vi "Query Frequency Mode.vi"(8 "error in (no error)":errorcluster, 10 "Channel (0: Channel 1)":T2 items=["Channel 1", "Channel 2"], 11 "VISA resource name":refnum<visa-resource-name>) -> (0 "error out":errorcluster, 1 "Mode (0: CW)":T1, 3 "VISA resource name out":refnum<visa-resource-name>)   [LabVIEW 2015, in "Tektronix AFG 3000 Series.lvlib"]
doc: "Queries the frequency mode (sweep vs. continuous) of a Tektronix AFG 3000 series function generator."
uses:
  Tektronix AFG 3000 Series.lvlib
  controls.llb/Channel.ctl
  controls.llb/Frequency Mode.ctl
  <vilib>/Utility/error.llb/DialogType.ctl
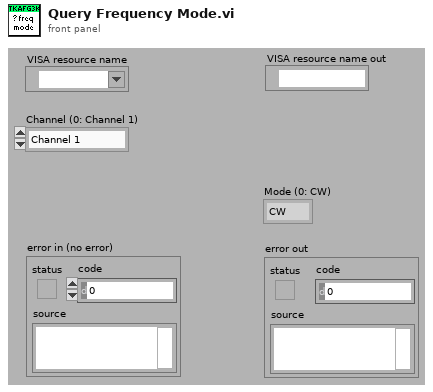
[diagram p1: front panel]
types:
  T1 = typedef "Frequency Mode.ctl" = enum16{"CW", "Sweep"}
  T2 = typedef "Channel.ctl" = u16
  T3 = typedef "DialogType.ctl" = u16
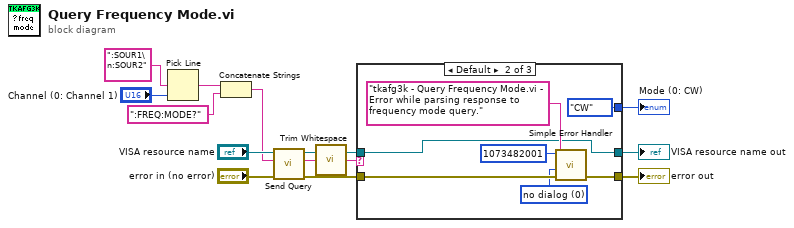
[diagram p0: block diagram]
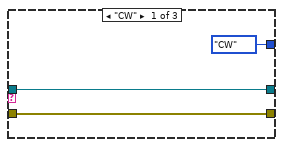
[diagram p2: hidden frame]
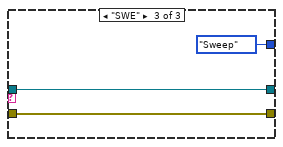
[diagram p3: hidden frame]
diagram:
  n1 = Pick Line(multi-line string=":SOUR1\n:SOUR2", line index="Channel (0: Channel 1)") -> (output string=w11:string)  [unwired: 1 out]
  n2 = Concatenate Strings(w11, ":FREQ:MODE?" ("format string")) -> (w10:string)
  n3 = call "Send Query.vi"("error in (no error)"="error in (no error)", "write buffer"=w10, "VISA resource name"="VISA resource name") -> ("error out"=w6:errorcluster, "read buffer"=w2:string, "VISA resource name out"=w5:refnum<visa-resource-name>)  [unwired: 1 in, 5 out]
  n4 = call <vilib>:"Trim Whitespace.vi"("string"=w2) -> ("trimmed string"=w1:string)  [unwired: 1 in]
  n5 = case shown="Default" w1 {
    tunnel: [Frequency_Mode."CW" ("Mode (0: CW) 2") Frequency_Mode."CW" ("Mode (0: CW) 2") Frequency_Mode."Sweep" ("Mode (0: CW) 2")] -> w7
    tunnel: w6 -> [w15 w23 w25]
    tunnel: w5 -> [w16 w18 w26]
    tunnel: [w16 w18 w26] -> w4
    tunnel: [w15 w22 w25] -> w3
    frame "CW" {
    }
    frame Default {
      w21 = T3 0 items=["no dialog", "OK message", "continue or stop message", "OK message + warnings", "continue/stop + warnings"] ("type of dialog (OK msg:1)")
      n6 = call <vilib>:"Simple Error Handler.vi"("error code (no error:0)"=1073482001, "error source (\" \")"="tkafg3k - Query Frequency Mode.vi - Error while parsing response to frequency mode query." ("error source (\" \")"), "type of dialog (OK msg:1)"=w21, "error in (no error)"=w23) -> ("error out"=w22:errorcluster)  [unwired: 5 out]
    }
    frame "SWE" {
    }
  }
  "error out" <- w3
  "VISA resource name out" <- w4
  "Mode (0: CW)" <- w7
